vi "ag33xxx - Close.vi"(8 "error in (no error)":errorcluster, 11 "VISA session":refnum<visa-resource-name>) -> (0 "error out":errorcluster)   [LabVIEW 2012]
doc: "This VI closes the I/O interface with the instrument."
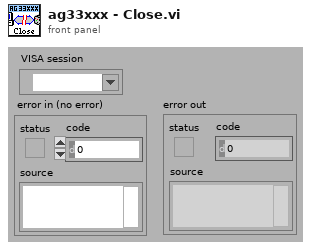
[diagram p1: front panel]
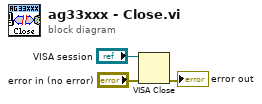
[diagram p0: block diagram]
diagram:
  n1 = VISA Close(VISA resource name="VISA session", error in (no error)="error in (no error)") -> (error out=→"error out":errorcluster)
